vi "niFpgaCompileFarm_Constants.vi"() -> ()   [LabVIEW 2017]
uses:
  <vilib>/rvi/CDR/niFpgaCompileFarm_ClientProtocols.ctl
panel:
  in  "Remote Protocol":T1=enum."2013 HTTP NI-Auth"
  in  "Local Protocol":T1=enum."2013 HTTP NI-Auth"
  in  "Cloud Protocol":T1=enum."2013 ni.com Services"
  in  "FPGAVendorId":string="ni.fpga"
  in  "LabVIEWProductId":string="labview.2017"
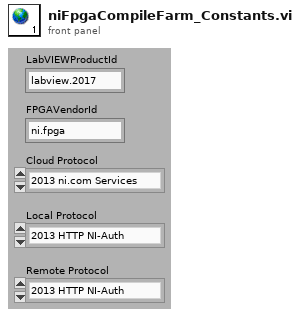
[diagram p1: front panel]
types:
  T1 = typedef "niFpgaCompileFarm_ClientProtocols.ctl" = enum16{"None", "Unsupported HTTP NI-Farm Authentication", "Unsupported HTTPS NI Farm Authentication", "2012 ni.com Services", "2012 HTTP NI-Auth", "2012 HTTPS NI-Auth", "2013 ni.com Services", "2013 HTTP NI-Auth", "2013 HTTPS NI-Auth"}
diagram:
